vi "Create Gradient Color by Start Color and End Color.vi"(8 "错误输入":errorcluster, 9 "Length":i32=256, 10 "End":u32(colorbox), 11 "Start":u32(colorbox)) -> (0 "错误输出":errorcluster, 3 "ColorArray":u32[](array[colorbox]))   [LabVIEW 2012, in "Picture Box Tools.lvlib"]
uses:
  <vilib>/Analysis/1siggen.llb/Ramp Pattern by Samples.vi
  Picture Box Tools.lvlib
  <vilib>/Analysis/NI_AALBase.lvlib
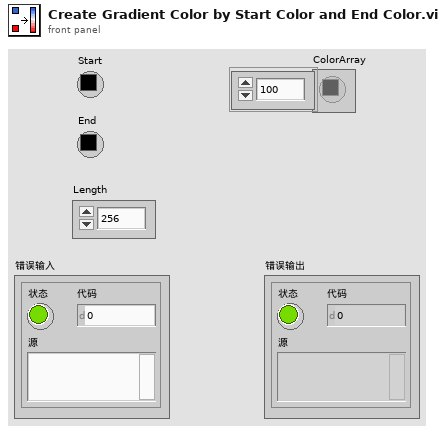
[diagram p1: front panel]
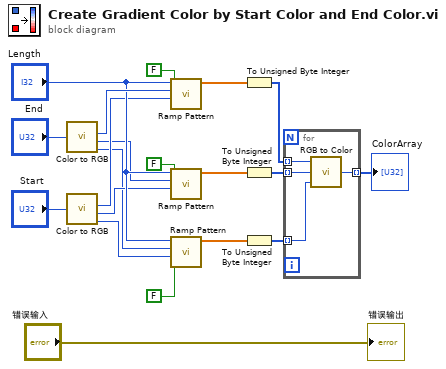
[diagram p0: block diagram]
diagram:
  n1 = call <vilib>:"Color to RGB.vi"("Color"="End") -> ("R"=w17:u8, "G"=w14:u8, "B"=w12:u8)  [unwired: 1 out]
  n2 = call <vilib>:"Color to RGB.vi"("Color"="Start") -> ("R"=w15:u8, "G"=w13:u8, "B"=w11:u8)  [unwired: 1 out]
  n3 = call-poly <vilib>:"Ramp Pattern.vi"("exclude end?"=FALSE, "start"=w15, "end"=w17, "samples"="Length") -> ("Ramp Pattern"=w10:dbl[])  [unwired: 6 in, 1 out]
  n4 = call-poly <vilib>:"Ramp Pattern.vi"("exclude end?"=FALSE, "start"=w13, "end"=w14, "samples"="Length") -> ("Ramp Pattern"=w9:dbl[])  [unwired: 6 in, 1 out]
  n5 = call-poly <vilib>:"Ramp Pattern.vi"("exclude end?"=FALSE, "start"=w11, "end"=w12, "samples"="Length") -> ("Ramp Pattern"=w8:dbl[])  [unwired: 6 in, 1 out]
  n6 = To Unsigned Byte Integer(number=w10) -> (unsigned 8bit integer=w7:u8[])
  n7 = To Unsigned Byte Integer(number=w9) -> (unsigned 8bit integer=w6:u8[])
  n8 = To Unsigned Byte Integer(number=w8) -> (unsigned 8bit integer=w5:u8[])
  n9 = for {
    tunnel: w7 -> [w24] mode=indexing
    tunnel: w6 -> [w23] mode=indexing
    tunnel: w5 -> [w22] mode=indexing
    tunnel: [w21] -> w4 mode=indexing
    n10 = call <vilib>:"RGB to Color.vi"("B"=w22, "G"=w23, "R"=w24) -> ("Color"=w21:u32)
  }
  "ColorArray" <- w4
  "错误输出" <- "错误输入"
